vi "Read Zero Point.vi"(8 "error in (no error)":errorcluster, 11 "VISA resource name":refnum<visa-resource-name>) -> (0 "error out":errorcluster, 1 "zero mode":bool, 2 "zero point":T1={"Capacitance"=0.0, "Loss"=0.0, "Frequency"=1000.0}, 3 "VISA resource name out":refnum<visa-resource-name>)   [LabVIEW 2020, in "Andeen-Hagerling 2700A.lvlib"]
doc: "Return the value of the zero point parameter and the whether or not zero mode is enabled."
uses:
  Andeen-Hagerling 2700A.lvlib
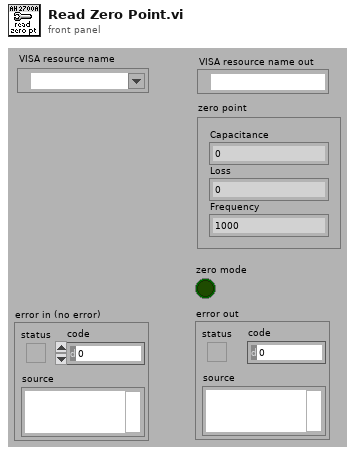
[diagram p1: front panel]
types:
  T1 = cluster{"Capacitance":dbl, "Loss":dbl, "Frequency":dbl}
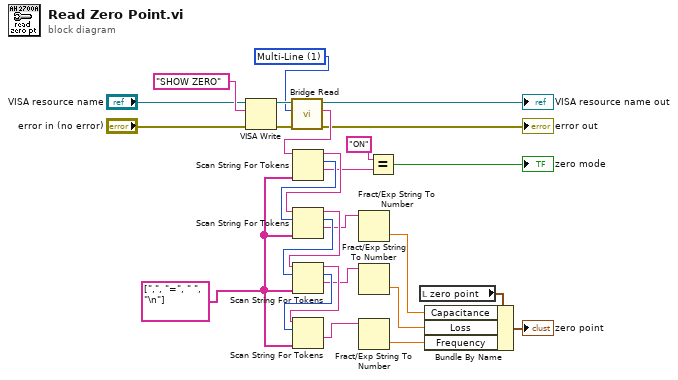
[diagram p0: block diagram]
diagram:
  w1 = u16 1 items=["Single Line", "Multi-Line"] ("Multiline")
  w6 = string[] [",", "=", " ", "\n"] ("delimiters (\\s,\\t,\\r,\\n)")
  n1 = VISA Write(VISA resource name="VISA resource name", write buffer="SHOW ZERO" ("string"), error in (no error)="error in (no error)") -> (VISA resource name out=w26:refnum<visa-resource-name>, error out=w25:errorcluster)  [unwired: 1 out]
  n2 = call "Bridge Read.vi"("error in (no error)"=w25, "multiline"=w1, "VISA resource name"=w26) -> ("error out"=→"error out":errorcluster, "read buffer"=w12:string, "VISA resource name out"=→"VISA resource name out":refnum<visa-resource-name>)  [unwired: 6 in]
  n3 = Scan String For Tokens(6:w6, 9:w12) -> (1:w9:string, 2:w11:i32, 3:w10:string)  [unwired: 4 in, 1 out]
  n4 = Scan String For Tokens(6:w6, 8:w11, 9:w10) -> (1:w15:string, 2:w23:i32, 3:w21:string)  [unwired: 3 in, 1 out]
  n5 = Scan String For Tokens(6:w6, 8:w23, 9:w21) -> (1:w20:string, 2:w24:i32, 3:w22:string)  [unwired: 3 in, 1 out]
  n6 = Scan String For Tokens(6:w6, 8:w24, 9:w22) -> (1:w19:string)  [unwired: 3 in, 3 out]
  n7 = Fract/Exp String To Number(string=w15) -> (number=w14:dbl)  [unwired: 3 in, 1 out]
  n8 = Fract/Exp String To Number(string=w20) -> (number=w17:dbl)  [unwired: 3 in, 1 out]
  n9 = Fract/Exp String To Number(string=w19) -> (number=w16:dbl)  [unwired: 3 in, 1 out]
  n10 = Equal?(x="ON", y=w9) -> (x = y?=→"zero mode":bool)
  n11 = local read "zero point"() -> (w18:T1)
  n12 = Bundle By Name(cluster=w18, "Capacitance"=w14, "Loss"=w17, "Frequency"=w16) -> (→"zero point":T1)
